vi "JKISM++ DebugTool Dialog.vi"() -> ()   [LabVIEW 2014, in "JKISM++ DebugTool.xnode"]
uses:
  JKISM++ DebugTool.xnode
panel:
  in  "Owning Application":refnum<vi>
  in  "Double Click To Run...":i32(listbox)=-1
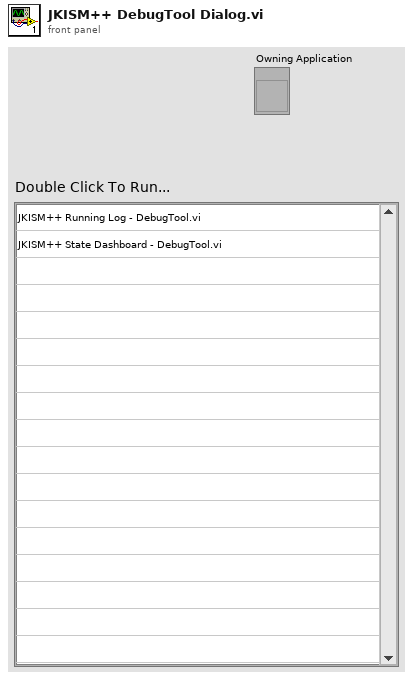
[diagram p1: front panel]
types:
  T1 = enum32{"Invalid", "Standard", "Closed", "Hidden", "Minimized", "Maximized"}
  T2 = enum32{"invalid app kind", "Development System", "Run Time System", "Student Edition", "Embedded LabVIEW", "Evaluation", "Custom"}
  T3 = cluster{"Core":cluster{"Current VI Reference":refnum<vi>, "Close Panel on Exit?":bool}, "Your Boolean data":bool, "ToolVIs":path[]}
  T4 = cluster{"Current VI Reference":refnum<vi>, "Close Panel on Exit?":bool}
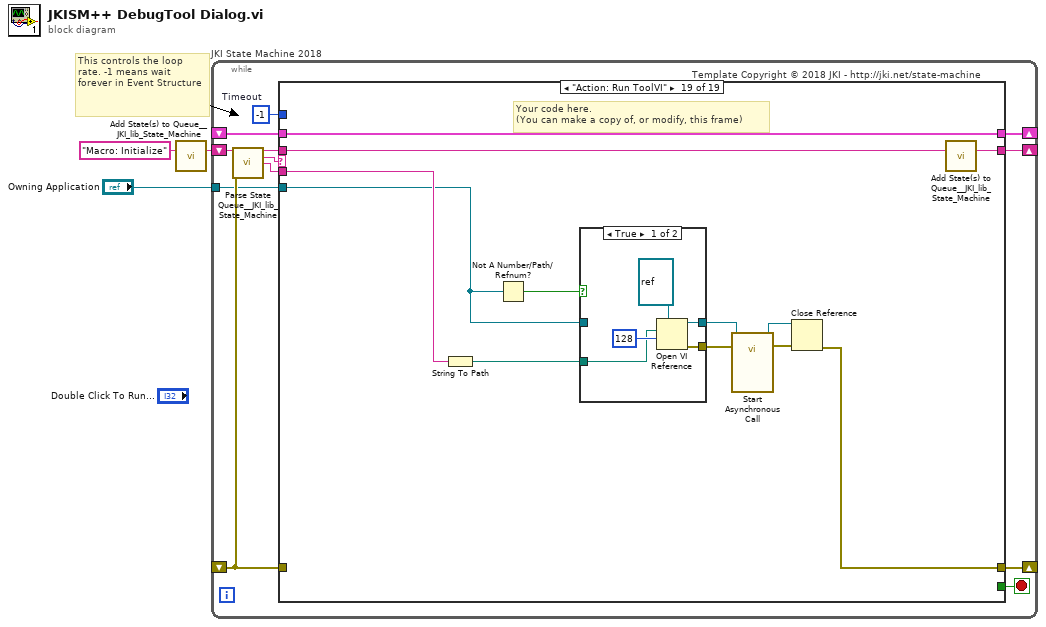
[diagram p0: block diagram]
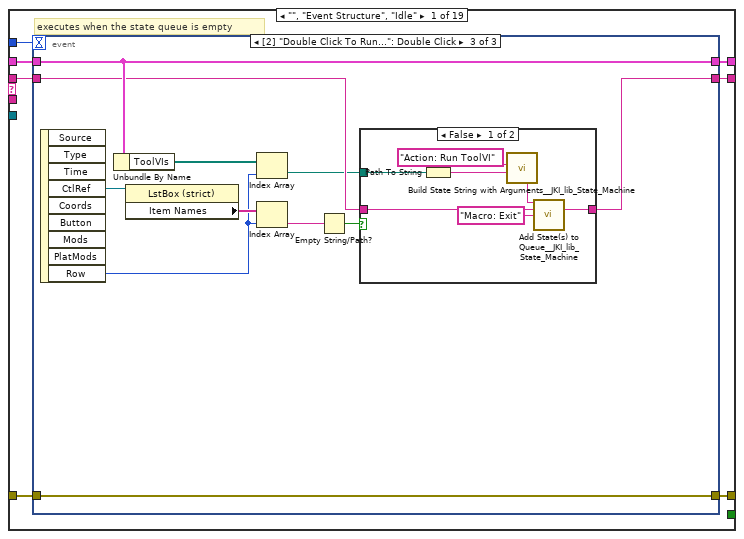
[diagram p2: hidden frame]
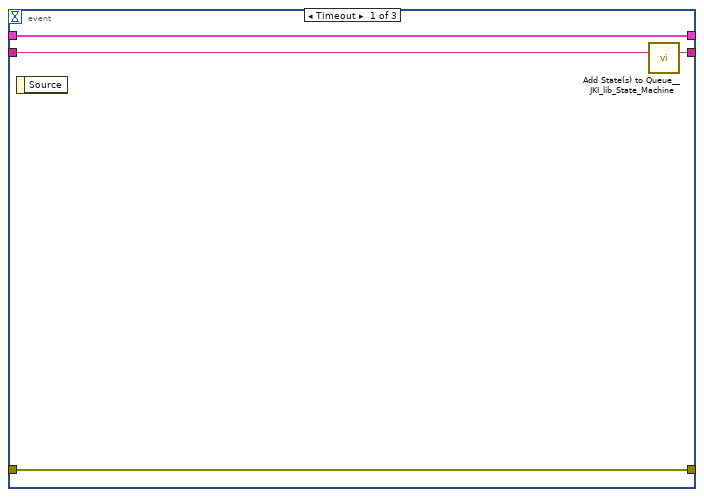
[diagram p3: hidden frame]
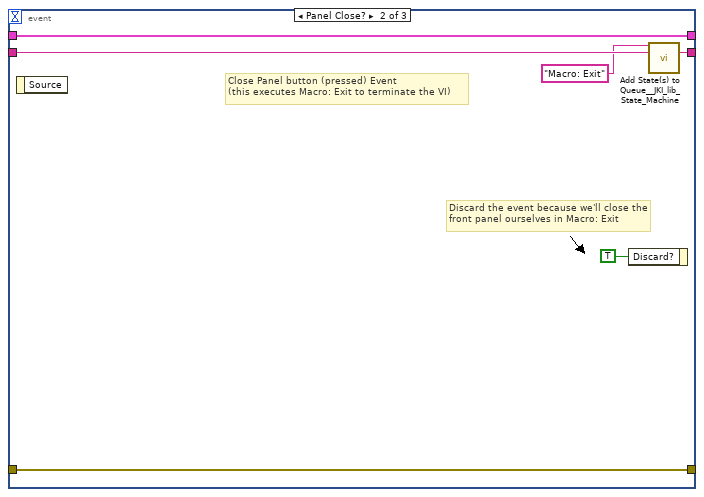
[diagram p4: hidden frame]
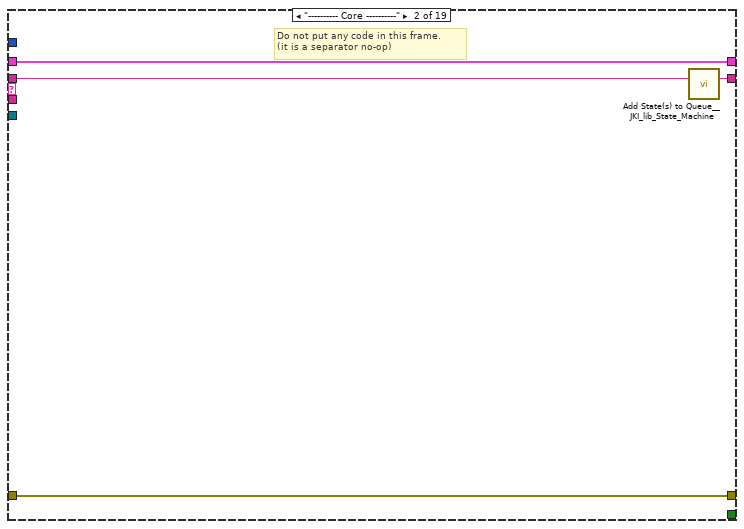
[diagram p6: hidden frame]
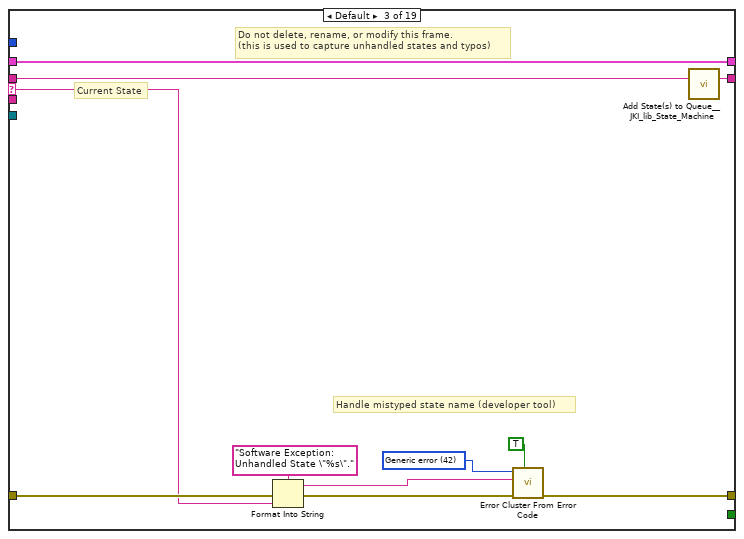
[diagram p7: hidden frame]
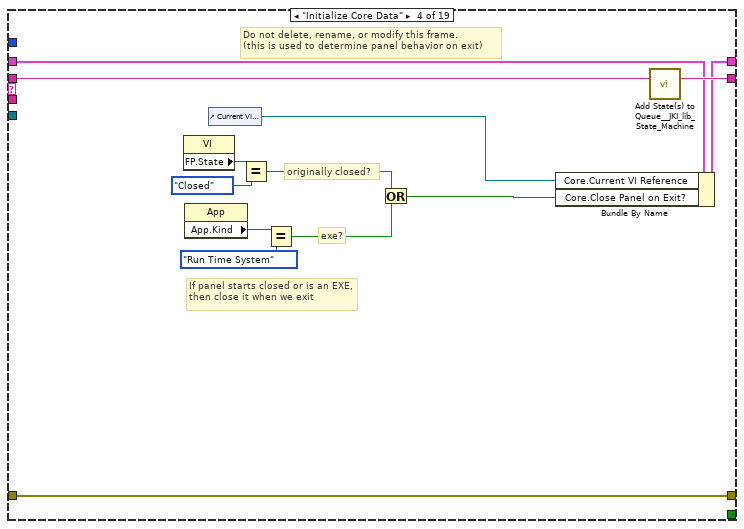
[diagram p8: hidden frame]
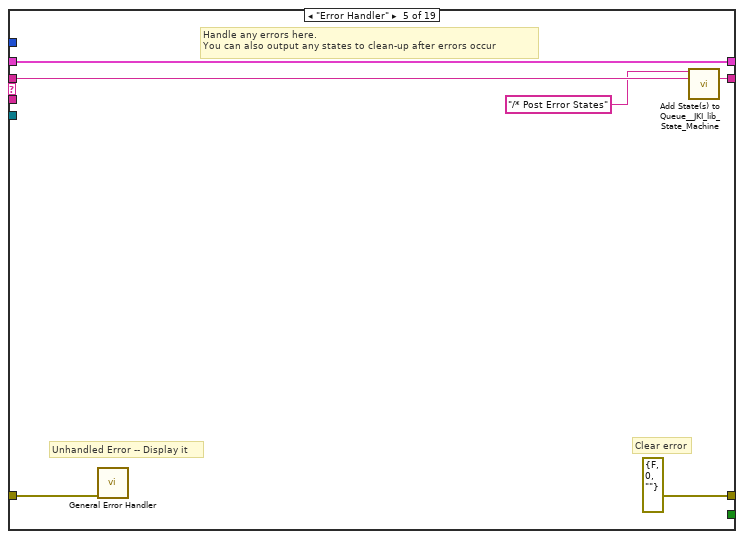
[diagram p9: hidden frame]
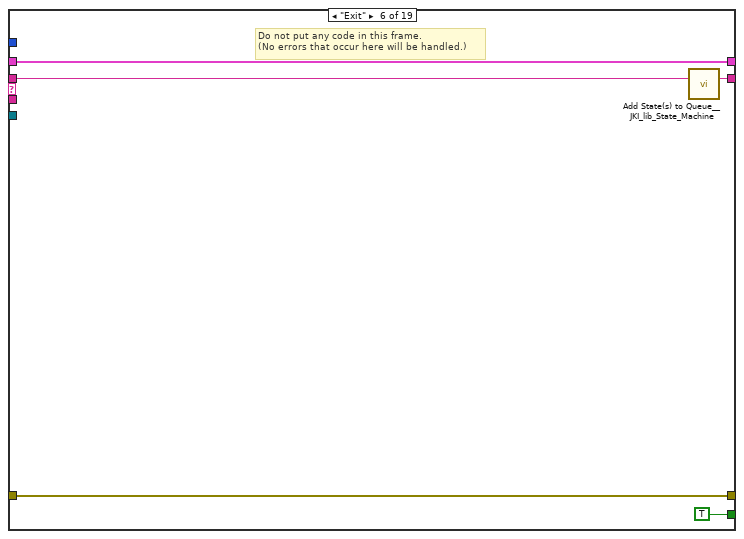
[diagram p10: hidden frame]
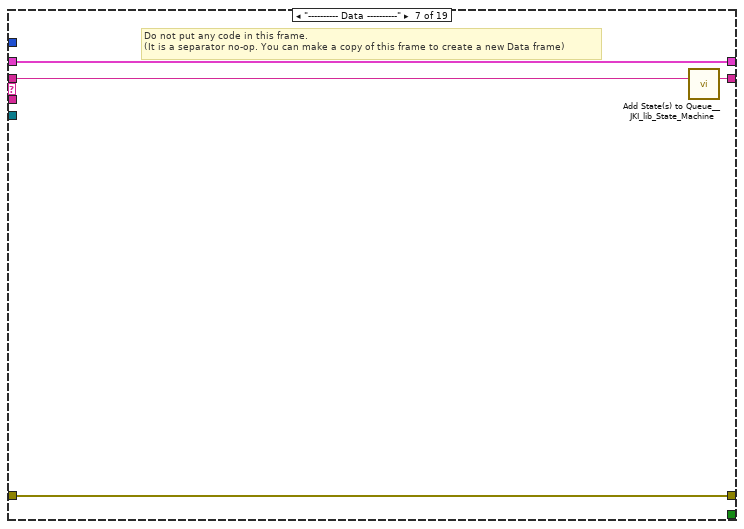
[diagram p11: hidden frame]
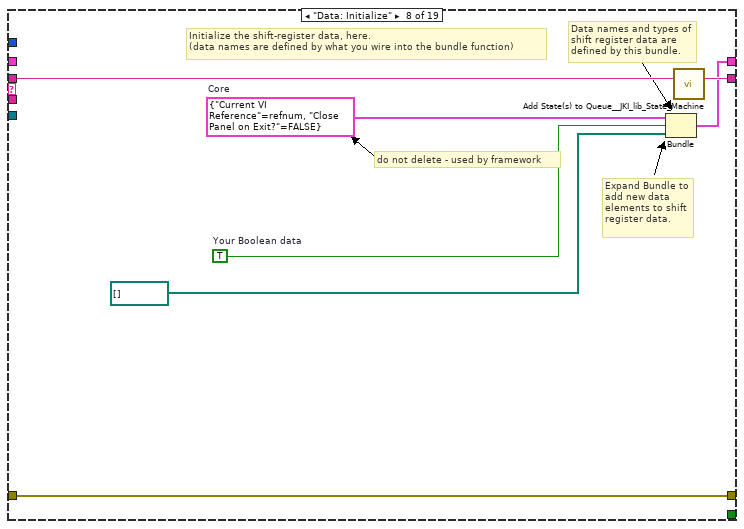
[diagram p12: hidden frame]
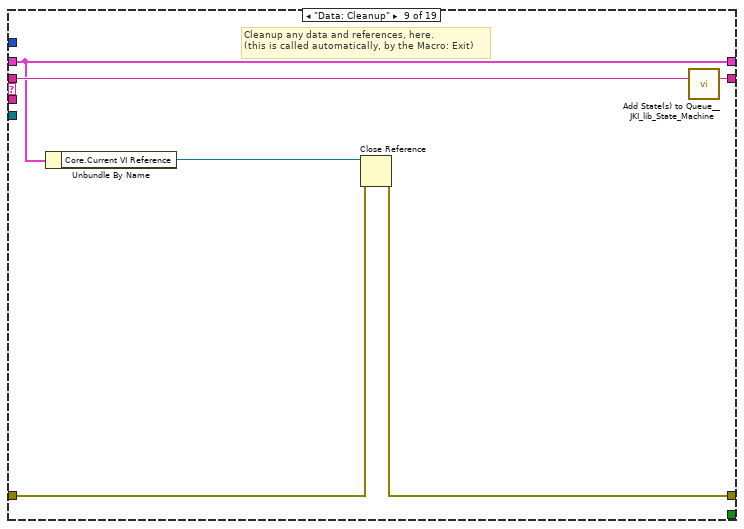
[diagram p13: hidden frame]
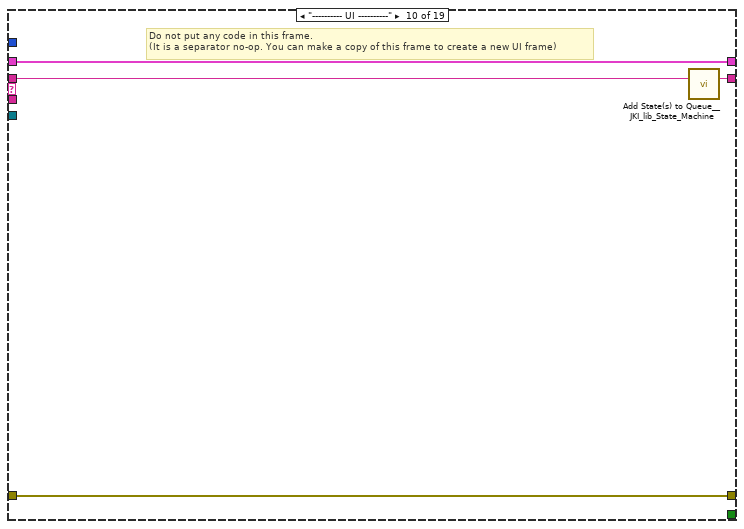
[diagram p14: hidden frame]
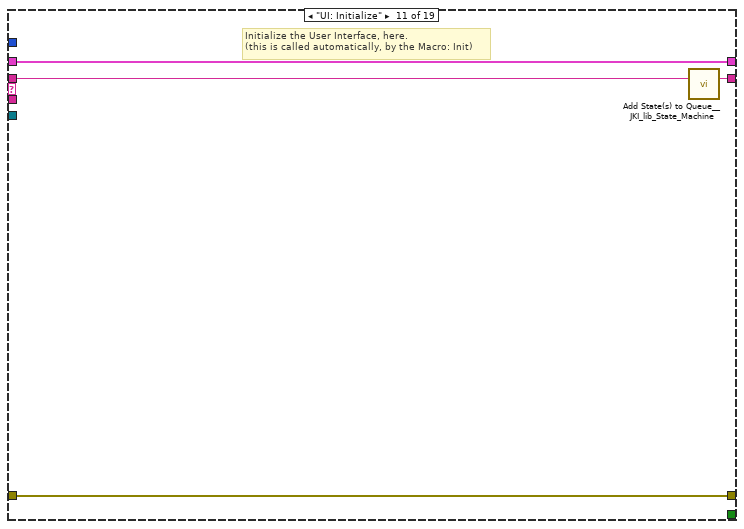
[diagram p15: hidden frame]
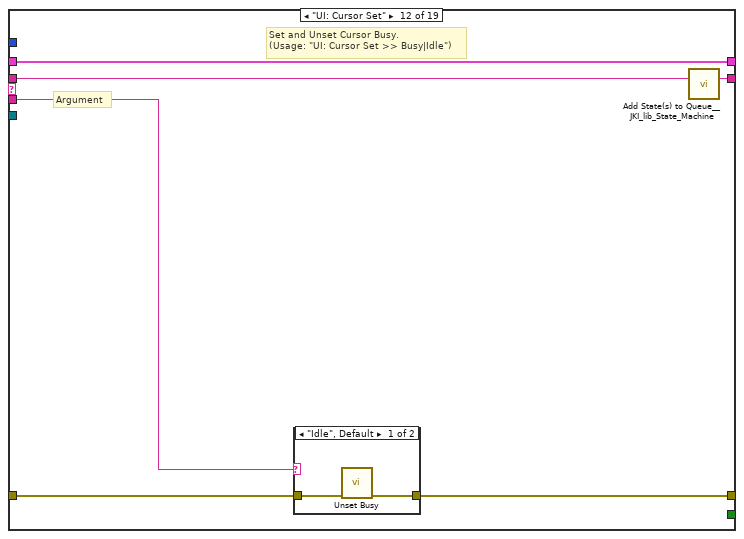
[diagram p16: hidden frame]
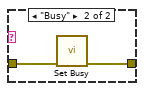
[diagram p17: hidden frame]
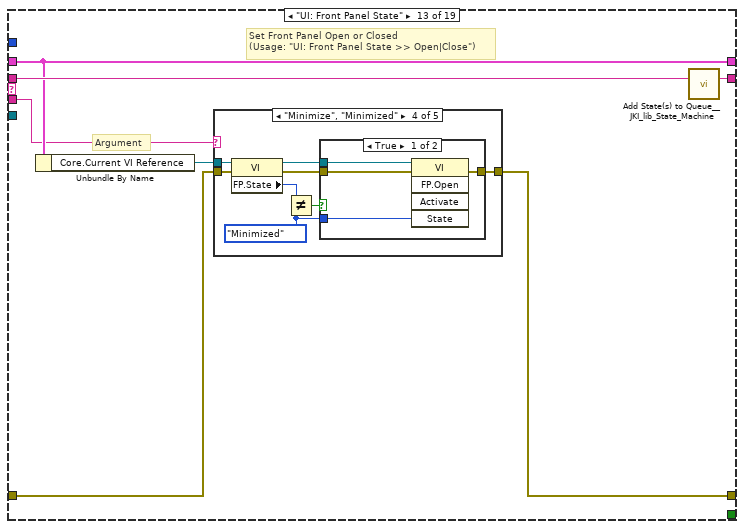
[diagram p18: hidden frame]
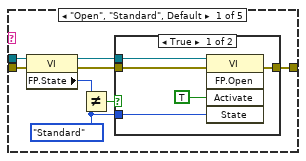
[diagram p19: hidden frame]
diagram:
  # "This controls the loop rate. -1 means wait forever in Event Structure"
  n1 = call <vilib>:"Add State(s) to Queue__JKI_lib_State_Machine.vi"("State(s) in (\"\")"="Macro: Initialize") -> ("States Out"=w3:string)  [unwired: 14 in]
  n2 = while "JKI State Machine 2018" {
    shift-right: [w8] -> _
    shift-left: _ -> [w7]
    shift-right: [w11] -> _
    shift-left: _ -> [w5]
    shift-right: [w10] -> _
    shift-left: w3 -> [w12]
    tunnel: "Owning Application" -> [w4]
    stop <- w9 stop-if-true
    w6 = -1  # Timeout
    # "Template Copyright © 2018 JKI - http://jki.net/state-machine"
    n3 = call <vilib>:"Parse State Queue__JKI_lib_State_Machine.vi"("State Queue"=w12, "Error In (no error)"=w5) -> ("Remaining States"=w14:string, "Current State"=w15:string, "Arguments"=w13:string)  [unwired: 11 in]
    n4 = case shown="\"Action: Run ToolVI\"" w15 {
      selector: w15 -> [_ _ w56 _ _ _ _ _ _ _ _ _ _ _ _ _ _ _ _]
      tunnel: w14 -> [w22 w55 w60 w79 w85 w90 w94 w101 w107 w111 w115 w121 w132 w208 w219 w224 w234 w238 w250]
      tunnel: w13 -> [_ _ _ _ _ _ _ _ _ _ _ w116 w126 _ _ _ _ _ w243]
      tunnel: w7 -> [w20 w52 w58 w72 w82 w88 w91 _ w102 w108 w113 w119 w128 w209 w216 w221 w231 w235 w248]
      tunnel: [w19 w53 w62 w76 errorcluster {"status"=FALSE, "code"=0, "source"=""} ("error out") w87 w92 w98 w103 w109 w112 w117 w129 w207 w217 w222 w232 w236 w239] -> w11
      tunnel: w5 -> [w18 w53 w61 w76 w81 w87 w92 w98 w104 w109 w112 w118 w130 w207 w217 w222 w232 w236 _]
      tunnel: [w21 w54 w59 w78 w84 w89 w93 w100 w106 w110 w114 w120 w131 w208 w218 w223 w233 w237 w249] -> w10
      tunnel: [_ _ _ _ _ TRUE _ _ _ _ _ _ _ _ _ _ _ _ _] -> w9
      tunnel: [w17 w52 w58 w77 w82 w88 w91 w99 w102 w108 w113 w119 w128 w200 w216 w221 w231 w235 w248] -> w8
      tunnel: w6 -> [w16 _ _ _ _ _ _ _ _ _ _ _ _ _ _ _ _ _ _]
      tunnel: w4 -> [_ _ _ _ _ _ _ _ _ _ _ _ _ _ _ _ _ _ w241]
      frame "", "Event Structure", "Idle" {
        # "executes when the state queue is empty"
        n5 = event shown="[2] \"Double Click To Run...\": Double Click" {
          selector: _ -> [_ _ _]
          dyn-events: _ -> [_ _ _]
          timeout: w16 -> [_ _ _]
          tunnel: w22 -> [w26 w32 w37]
          tunnel: [w25 w31 w36] -> w21
          tunnel: w20 -> [w23 w29 w40]
          tunnel: [w24 w30 w43] -> w19
          tunnel: w18 -> [w24 w30 w43]
          tunnel: [w23 w29 w40] -> w17
          event Timeout {
            n6 = event-data() -> ()  [unwired: 1 in, 1 out]
            n7 = call <vilib>:"Add State(s) to Queue__JKI_lib_State_Machine.vi"("State(s) in (\"\")"=w26) -> ("States Out"=w25:string)  [unwired: 14 in]
          }
          event Panel Close? {
            # "Discard the event because we'll close the front panel ourselves in Macro: Exit"
            # "Close Panel button (pressed) Event\n(this executes Macro: Exit to terminate the VI)"
            n8 = event-data() -> ()  [unwired: 1 in, 1 out]
            n9 = event-data("Discard?"=TRUE) -> ()  [unwired: 1 in, 1 out]
            n10 = call <vilib>:"Add State(s) to Queue__JKI_lib_State_Machine.vi"("State(s) in Front (\"\")"="Macro: Exit", "State(s) in (\"\")"=w32) -> ("States Out"=w31:string)  [unwired: 13 in]
          }
          event "Double Click To Run...": Double Click {
            n11 = event-data() -> ("CtlRef"=w42:refnum<vi>, "Row"=w38:i32)  [unwired: 1 in, 7 out]
            n12 = Unbundle By Name(w40) -> ("ToolVIs"=w39:path[])
            n13 = property class="LstBox (strict)"(reference=w42) -> ("Item Names"=w41:string[])  [unwired: 1 in, 2 out]
            n14 = Index Array(array=w39, index=w38) -> (element=w33:path)
            n15 = Index Array(array=w41, index=w38) -> (element=w35:string)
            n16 = Empty String/Path?(string/path=w35) -> (empty?=w34:bool)
            n17 = case shown="False" w34 {
              tunnel: w37 -> [w50 w51]
              tunnel: [w49 w51] -> w36
              tunnel: w33 -> [w46 _]
              frame False {
                n18 = Path To String(path=w46) -> (string=w44:string)
                n19 = call <vilib>:"Build State String with Arguments__JKI_lib_State_Machine.vi"("Arguments (\"\")"=w44, "State"="Action: Run ToolVI") -> ("State with Arguments"=w47:string)  [unwired: 4 in]
                n20 = call <vilib>:"Add State(s) to Queue__JKI_lib_State_Machine.vi"("State(s) in Front (\"\")"=w47, "State(s) in (\"\")"=w50, "State(s) at Back (\"\")"="Macro: Exit" ("State(s) at Back (\"\")")) -> ("States Out"=w49:string)  [unwired: 12 in]
              }
              frame True {
              }
            }
          }
        }
      }
      frame "---------- Core ----------" {
        # "Do not put any code in this frame.\n(it is a separator no-op)"
        n21 = call <vilib>:"Add State(s) to Queue__JKI_lib_State_Machine.vi"("State(s) in (\"\")"=w55) -> ("States Out"=w54:string)  [unwired: 14 in]
      }
      frame Default {
        w65 = 42 items=["No error", "Argument error", "Memory is full", "Out of zone", "End of file", "File already open", "Generic file I/O error", "File not found", "File permission error", "Disk is full", "Duplicate path", "Too many files open", "System feature not enabled", "Resource file not found", "Cannot add resource", "Resource not found", "Image not found", "Image memory error", "Pen does not exist", "Config type invalid", "Config token not found", "Config parse error", "Config memory error", "Bad external code format", "Bad external code offset", "External code not present", "Null window", "Destroy window error", "Null menu", "Print aborted", "Bad print record", "Print driver error", "Windows error during printing", "Memory error during printing", "Print dialog error", "Generic print error", "Invalid device refnum", "Device not found", "Device parameter error", "Device unit error", "Cannot open device", "Device call aborted", "Generic error", "Cancelled by user", "Object ID too low", "Object ID too high", "Object not in heap", "Unknown heap", "Unknown object (invalid DefProc)", "Unknown object (DefProc not in table)", "Message out of range", "Invalid (null) method", "Unknown message", "Manager call not supported", "Bad address", "Network operation in progress", "Network operation timed out", "Connection is busy", "Network attribute not supported", "Network error", "Address in use", "System out of memory", "Connection aborted", "Connection refused", "Not connected", "Already connected", "Connection closed", "Initialization error (interapplication manager)", "Bad occurrence", "Wait on unbound occurrence handler", "Occurrence queue overflow", "Datalog type conflict", "Unused", "Unrecognized type (interapplication manager)", "Memory corrupt", "Failed to make temporary DLL", "Old CIN version", "Drag socket not found", "Failed to load drop-object", "Failed to register OLE object", "Failed to release OLE object", "Format specifier type mismatch", "Unknown format specifier", "Too few format specifiers", "Too many format specifiers", "Scan failed", "Newer CIN version", "Error converting to variant", "Runtime menu error", "Password tampered", "Variant attribute not found", "Incompatible variant data type", "Event data is not available", "Event Store is not present", "Occurrence is not found", "Event Queue is not created", "Event info is not available", "Refnum passed is NULL", "Error retrieving Class GUID", "Error retrieving CoClass GUID", "Error retrieving TypeLib GUID.", "Bad built application magic bytes.", "Specific driver is different from the specific driver associated with the Logical Name.", "There is no session opened to the class driver.", "Max Error", "MAX - Error with config objects", "MAX - Error loading configuration", "MAX - Group not supported"]
        # "Current State"
        # "Do not delete, rename, or modify this frame.\n(this is used to capture unhandled states and typos)"
        # "Handle mistyped state name (developer tool)"
        n22 = Format Into String(format string="Software Exception: Unhandled State \"%s\"." ("message"), error in=w61, w56) -> (resulting string=w64:string, error out=w63:errorcluster)  [unwired: 1 in]
        n23 = call <vilib>:"Error Cluster From Error Code.vi"("show call chain? (False)"=TRUE, "error in (no error)"=w63, "error message (\"\")"=w64, "error code (0)"=w65) -> ("error out"=w62:errorcluster)  [unwired: 5 in]
        n24 = call <vilib>:"Add State(s) to Queue__JKI_lib_State_Machine.vi"("State(s) in (\"\")"=w60) -> ("States Out"=w59:string)  [unwired: 14 in]
      }
      frame "Initialize Core Data" {
        # "Do not delete, rename, or modify this frame.\n(this is used to determine panel behavior on exit)"
        # "originally closed?"
        # "exe?"
        # "If panel starts closed or is an EXE, then close it when we exit"
        n25 = property class="VI"() -> ("FP.State"=w69:T1)  [unwired: 2 in, 2 out]
        n26 = property class="App"() -> ("App.Kind"=w75:T2)  [unwired: 2 in, 2 out]
        n27 = control-ref of="Current VI Reference"() -> (w70:refnum<vi>)
        n28 = Equal?(x=w69, y=T1."Closed" ("Front Panel Window:State")) -> (x = y?=w67:bool)
        n29 = Equal?(x=w75, y=T2."Run Time System" ("Application:Kind")) -> (x = y?=w73:bool)
        n30 = Or(x=w67, y=w73) -> (x .or. y?=w71:bool)
        n31 = Bundle By Name(cluster=w72, "Core.Current VI Reference"=w70, "Core.Close Panel on Exit?"=w71) -> (w77:T3)
        n32 = call <vilib>:"Add State(s) to Queue__JKI_lib_State_Machine.vi"("State(s) in (\"\")"=w79) -> ("States Out"=w78:string)  [unwired: 14 in]
      }
      frame "Error Handler" {
        # "Unhandled Error -- Display it"
        # "Handle any errors here.\nYou can also output any states to clean-up after errors occur"
        # "Clear error"
        n33 = call <vilib>:"General Error Handler.vi"("error in (no error)"=w81) -> ()  [unwired: 10 in, 5 out]
        n34 = call <vilib>:"Add State(s) to Queue__JKI_lib_State_Machine.vi"("State(s) in Front (\"\")"="/* Post Error States", "State(s) in (\"\")"=w85) -> ("States Out"=w84:string)  [unwired: 13 in]
      }
      frame "Exit" {
        # "Do not put any code in this frame.\n(No errors that occur here will be handled.)"
        n35 = call <vilib>:"Add State(s) to Queue__JKI_lib_State_Machine.vi"("State(s) in (\"\")"=w90) -> ("States Out"=w89:string)  [unwired: 14 in]
      }
      frame "---------- Data ----------" {
        # "Do not put any code in this frame.\n(It is a separator no-op. You can make a copy of this frame to create a new Data frame)"
        n36 = call <vilib>:"Add State(s) to Queue__JKI_lib_State_Machine.vi"("State(s) in (\"\")"=w94) -> ("States Out"=w93:string)  [unwired: 14 in]
      }
      frame "Data: Initialize" {
        w96 = T4 {"Current VI Reference"=refnum, "Close Panel on Exit?"=FALSE}  # Core
        w97 = TRUE  # Your Boolean data
        # "do not delete - used by framework"
        # "Expand Bundle to add new data elements to shift register data."
        # "Data names and types of shift register data are defined by this bundle."
        # "Initialize the shift-register data, here.\n(data names are defined by what you wire into the bundle function)"
        n37 = Bundle("Core"=w96, "Your Boolean data"=w97, "ToolVIs"=path[] []) -> (w99:T3)  [unwired: 1 in]
        n38 = call <vilib>:"Add State(s) to Queue__JKI_lib_State_Machine.vi"("State(s) in (\"\")"=w101) -> ("States Out"=w100:string)  [unwired: 14 in]
      }
      frame "Data: Cleanup" {
        # "Cleanup any data and references, here.\n(this is called automatically, by the Macro: Exit)"
        n39 = Unbundle By Name(w102) -> ("Core.Current VI Reference"=w105:refnum<vi>)
        n40 = Close Reference(reference=w105, error in (no error)=w104) -> (error out=w103:errorcluster)
        n41 = call <vilib>:"Add State(s) to Queue__JKI_lib_State_Machine.vi"("State(s) in (\"\")"=w107) -> ("States Out"=w106:string)  [unwired: 14 in]
      }
      frame "---------- UI ----------" {
        # "Do not put any code in this frame.\n(It is a separator no-op. You can make a copy of this frame to create a new UI frame)"
        n42 = call <vilib>:"Add State(s) to Queue__JKI_lib_State_Machine.vi"("State(s) in (\"\")"=w111) -> ("States Out"=w110:string)  [unwired: 14 in]
      }
      frame "UI: Initialize" {
        # "Initialize the User Interface, here.\n(this is called automatically, by the Macro: Init)"
        n43 = call <vilib>:"Add State(s) to Queue__JKI_lib_State_Machine.vi"("State(s) in (\"\")"=w115) -> ("States Out"=w114:string)  [unwired: 14 in]
      }
      frame "UI: Cursor Set" {
        # "Argument"
        # "Set and Unset Cursor Busy.\n(Usage: \"UI: Cursor Set >> Busy|Idle\")"
        n44 = case shown="\"Idle\", Default" w116 {
          tunnel: w118 -> [w123 w125]
          tunnel: [w122 w124] -> w117
          frame "Idle", Default {
            n45 = call <vilib>:"Unset Busy.vi"("error in (no error)"=w123) -> ("error out"=w122:errorcluster)  [unwired: 10 in]
          }
          frame "Busy" {
            n46 = call <vilib>:"Set Busy.vi"("error in (no error)"=w125) -> ("error out"=w124:errorcluster)  [unwired: 9 in, 1 out]
          }
        }
        n47 = call <vilib>:"Add State(s) to Queue__JKI_lib_State_Machine.vi"("State(s) in (\"\")"=w121) -> ("States Out"=w120:string)  [unwired: 14 in]
      }
      frame "UI: Front Panel State" {
        # "Argument"
        # "Set Front Panel Open or Closed\n(Usage: \"UI: Front Panel State >> Open|Close\")"
        n48 = Unbundle By Name(w128) -> ("Core.Current VI Reference"=w127:refnum<vi>)
        n49 = case shown="\"Minimize\", \"Minimized\"" w126 {
          tunnel: w130 -> [w138 w153 w164 w177 w190]
          tunnel: [w140 w154 w166 w179 w192] -> w129
          tunnel: w127 -> [w139 w151 w165 w178 w191]
          frame "Open", "Standard", Default {
            w133 = T1."Standard" ("State")
            n50 = property class="VI"(reference=w139, error in=w138) -> (reference out=w136:refnum<vi>, error out=w137:errorcluster, "FP.State"=w135:T1)
            n51 = Not Equal?(x=w135, y=w133) -> (x != y?=w134:bool)
            n52 = case shown="True" w134 {
              tunnel: [w144 w146] -> w140
              tunnel: w137 -> [w143 w146]
              tunnel: w136 -> [w142 _]
              tunnel: w133 -> [w141 _]
              frame True {
                n53 = invoke class="VI" method="FP.Open"(reference=w142, error in=w143, "Activate"=TRUE, "State"=w141) -> (error out=w144:errorcluster)  [unwired: 1 in, 4 out]
              }
              frame False {
              }
            }
          }
          frame "Close", "Closed" {
            n54 = property class="VI"(reference=w151, error in=w153) -> (reference out=w150:refnum<vi>, error out=w152:errorcluster, "FP.State"=w148:T1)
            n55 = Not Equal?(x=w148, y=T1."Closed" ("Front Panel Window:State")) -> (x != y?=w147:bool)
            n56 = case shown="True" w147 {
              tunnel: [w155 w158] -> w154
              tunnel: w152 -> [w155 w157]
              tunnel: w150 -> [_ w156]
              frame False {
              }
              frame True {
                n57 = invoke class="VI" method="FP.Close"(reference=w156, error in=w157) -> (error out=w158:errorcluster)  [unwired: 1 in, 2 out]
              }
            }
          }
          frame "Hidden", "Hide" {
            w159 = T1."Hidden" ("State")
            n58 = property class="VI"(reference=w165, error in=w164) -> (reference out=w162:refnum<vi>, error out=w163:errorcluster, "FP.State"=w161:T1)
            n59 = Not Equal?(x=w161, y=w159) -> (x != y?=w160:bool)
            n60 = case shown="True" w160 {
              tunnel: [w170 w171] -> w166
              tunnel: w163 -> [w169 w171]
              tunnel: w162 -> [w168 _]
              tunnel: w159 -> [w167 _]
              frame True {
                n61 = invoke class="VI" method="FP.Open"(reference=w168, error in=w169, "State"=w167) -> (error out=w170:errorcluster)  [unwired: 2 in, 4 out]
              }
              frame False {
              }
            }
          }
          frame "Minimize", "Minimized" {
            w172 = T1."Minimized" ("State")
            n62 = property class="VI"(reference=w178, error in=w177) -> (reference out=w175:refnum<vi>, error out=w176:errorcluster, "FP.State"=w174:T1)
            n63 = Not Equal?(x=w174, y=w172) -> (x != y?=w173:bool)
            n64 = case shown="True" w173 {
              tunnel: [w183 w184] -> w179
              tunnel: w176 -> [w182 w184]
              tunnel: w175 -> [w181 _]
              tunnel: w172 -> [w180 _]
              frame True {
                n65 = invoke class="VI" method="FP.Open"(reference=w181, error in=w182, "State"=w180) -> (error out=w183:errorcluster)  [unwired: 2 in, 4 out]
              }
              frame False {
              }
            }
          }
          frame "Maximize", "Maximized" {
            w185 = T1."Maximized" ("State")
            n66 = property class="VI"(reference=w191, error in=w190) -> (reference out=w188:refnum<vi>, error out=w189:errorcluster, "FP.State"=w187:T1)
            n67 = Not Equal?(x=w187, y=w185) -> (x != y?=w186:bool)
            n68 = case shown="True" w186 {
              tunnel: [w196 w197] -> w192
              tunnel: w189 -> [w195 w197]
              tunnel: w188 -> [w194 _]
              tunnel: w185 -> [w193 _]
              frame True {
                n69 = invoke class="VI" method="FP.Open"(reference=w194, error in=w195, "State"=w193) -> (error out=w196:errorcluster)  [unwired: 2 in, 4 out]
              }
              frame False {
              }
            }
          }
        }
        n70 = call <vilib>:"Add State(s) to Queue__JKI_lib_State_Machine.vi"("State(s) in (\"\")"=w132) -> ("States Out"=w131:string)  [unwired: 14 in]
      }
      frame "UI: Update List" {
        n71 = Current VI's Path() -> (path=w206:path)
        n72 = Strip Path(path=w206) -> (stripped path=w205:path)  [unwired: 1 out]
        n73 = Strip Path(path=w205) -> (stripped path=w204:path)  [unwired: 1 out]
        n74 = List Folder(path=w204, pattern="*.vi") -> (path out=w201:path, filenames=w202:string[])  [unwired: 2 in, 2 out]
        n75 = for {
          tunnel: w202 -> [w211] mode=indexing
          tunnel: w201 -> [w214]
          tunnel: [w213] -> w199 mode=indexing if=w210
          tunnel: [w211] -> w198 mode=indexing if=w210
          n76 = Match Pattern(string=w211, regular expression="^_") -> (offset past match=w212:i32)  [unwired: 1 in, 3 out]
          n77 = Less Than 0?(x=w212) -> (x < 0?=w210:bool)
          n78 = Build Path(base path=w214, name or relative path=w211) -> (appended path=w213:path)
        }
        n79 = property on="Double Click To Run..." class="LstBox (strict)"("Item Names"=w198) -> ()  [unwired: 2 in, 2 out]
        n80 = Bundle By Name(cluster=w209, "ToolVIs"=w199) -> (w200:T3)
      }
      frame "---------- Macro ----------" {
        # "Do not put any code in this frame.\n(It is a separator no-op. You can make a copy of this frame to create a new Macro frame)"
        n81 = call <vilib>:"Add State(s) to Queue__JKI_lib_State_Machine.vi"("State(s) in (\"\")"=w219) -> ("States Out"=w218:string)  [unwired: 14 in]
      }
      frame "Macro: Initialize" {
        w220 = "Data: Initialize\nInitialize Core Data\nUI: Initialize\nUI: Front Panel State >> Open\nUI: Update List"  # Data: Initialize Initialize Core Data UI: Initialize UI: Front Panel State >> Open UI: Update List
        # "Initialization Macro\n(This is called once, when the VI starts)"
        n82 = call <vilib>:"Add State(s) to Queue__JKI_lib_State_Machine.vi"("State(s) in Front (\"\")"=w220, "State(s) in (\"\")"=w224) -> ("States Out"=w223:string)  [unwired: 13 in]
      }
      frame "Macro: Exit" {
        # "Exit Macro\n(This is called once, when the VI exits)"
        n83 = Unbundle By Name(w231) -> ("Core.Close Panel on Exit?"=w230:bool)
        n84 = Select(t="UI: Front Panel State >> Close", s=w230, f="") -> (s? t:f=w227:string)
        n85 = call <vilib>:"Add State(s) to Queue__JKI_lib_State_Machine.vi"("State(s) in (\"\")"=w227, "State(s) at Back (\"\")"="Data: Cleanup\nExit") -> ("States Out"=w225:string)  [unwired: 13 in]
        n86 = call <vilib>:"Add State(s) to Queue__JKI_lib_State_Machine.vi"("State(s) in Front (\"\")"=w225, "State(s) in (\"\")"=w234) -> ("States Out"=w233:string)  [unwired: 13 in]
      }
      frame "---------- Action ----------" {
        # "Template Separator\n(You can make a copy of, or modify, this frame)"
        n87 = call <vilib>:"Add State(s) to Queue__JKI_lib_State_Machine.vi"("State(s) in (\"\")"=w238) -> ("States Out"=w237:string)  [unwired: 14 in]
      }
      frame "Action: Run ToolVI" {
        # "Your code here.\n(You can make a copy of, or modify, this frame)"
        n88 = String To Path(string=w243) -> (path=w242:path)
        n89 = Not A Number/Path/Refnum?(number/path/refnum=w241) -> (NaN/Path/Refnum?=w240:bool)
        n90 = case shown="True" w240 {
          tunnel: [w254 w260] -> w245
          tunnel: [w253 w259] -> w244
          tunnel: w242 -> [w251 w257]
          tunnel: w241 -> [_ w256]
          frame True {
            n91 = Open VI Reference(type specifier VI Refnum (for type only)=refnum<vi> refnum, vi path=w251, options=128) -> (vi reference=w254:refnum<vi>, error out=w253:errorcluster)  [unwired: 3 in]
          }
          frame False {
            n92 = Open VI Reference(type specifier VI Refnum (for type only)=refnum<vi> refnum, application reference (local)=w256, vi path=w257, options=128) -> (vi reference=w260:refnum<vi>, error out=w259:errorcluster)  [unwired: 2 in]
          }
        }
        n93 = call-by-ref "Start Asynchronous Call"(reference=w245, error in=w244) -> (reference out=w247:refnum<vi>, error out=w246:errorcluster)  [unwired: 12 in]
        n94 = Close Reference(reference=w247, error in (no error)=w246) -> (error out=w239:errorcluster)
        n95 = call <vilib>:"Add State(s) to Queue__JKI_lib_State_Machine.vi"("State(s) in (\"\")"=w250) -> ("States Out"=w249:string)  [unwired: 14 in]
      }
    }
  }
